vi "CTRE_CANTalonSRX_GetParameter.vi"(8 "error in (no error)":errorcluster, 10 "Parameter":T1=1 items=["Slot 0 - P"=1, "Slot 0 - I"=2, "Slot 0 - D"=3, "Slot 0 - F"=4, "Slot 0 - I Zone"=5, "Slot 0 - Ramp Rate"=6, "Slot 1 - P"=11, "Slot 1 - I"=12, "Slot 1 - D"=13, "Slot 1 - F"=14, "Slot 1 - I Zone"=15, "Slot 1 - Ramp Rate"=16, "Soft Limit - Forward"=21, "Soft Limit - Reverse"=22, "Soft Limit - Forward Enable"=23, "Soft Limit - Reverse Enable"=24, "On Boot - Brake Mode"=31, "On Boot - Limit Normally Closed - Forward"=32, "On Boot - Limit Normally Closed - Reverse"=33, "On Boot - Limit Disabled - Forward"=34, "On Boot - Limit Disabled - Reverse"=35, "Fault - Over Temp"=41, "Fault - Under Voltage"=42, "Fault - Forward Limit"=43, "Fault - Reverse Limit"=44, "Fault - Hardware Failure"=45, "Fault - Forward Soft Limit"=46, "Fault - Reverse Soft Limit"=47, "Sticky Fault - Over Temp"=48, "Sticky Fault - Under Voltage"=49, "Sticky Fault - Forward Limit"=50, "Sticky Fault - Reverse Limit"=51, "Sticky Fault - Forward Soft Limit"=52, "Sticky Fault - Reverse Soft Limit"=53, "Applied Throttle"=61, "Closed-Loop Error"=62, "Select Feedback Device"=63, "Reverse Closed-Loop Output"=64, "Mode Select"=65, "Profile Slot Select"=66, "Ramp Throttle"=67, "Reverse Feedback Sensor"=68, "Limit Switch Enabled"=69, "Limit Switch Closed - Forward"=70, "Limit Switch Closed - Reverse"=71, "Sensor Position"=73, "Sensor Velocity"=74, "Current"=75, "Brake is Enabled"=76, "Encoder Position"=77, "Encoder Velocity"=78, "Encoder Index Rise Events"=79, "Encoder A Pin State"=80, "Encoder B Pin State"=81, "Encoder Index Pin State"=82, "Analog In with Overflow"=83, "Analog In Velocity"=84, "Temperature"=85, "Battery Voltage"=86, "Reset Count"=87, "Reset Flags"=88, "Firmware Version"=89, "Settings Changed"=90, "Quad Filter Enable"=91, "Ignore Disable Broadcast"=92, "I Accumulator"=93, "Status 1 Frame Rate Ms"=94, "Status 2 Frame Rate Ms"=95, "Status 3 Frame Rate Ms"=96, "Status 4 Frame Rate Ms"=97, "Status 6 Frame Rate Ms"=98, "Status 7 Frame Rate Ms"=99, "Enable Index Pin Clear Position"=100, "Peak Positive Output"=104, "Nominal Positive Output"=105, "Peak Negative Output"=106, "Nominal Negative Output"=107, "Quad Index Pin Polarity"=108, "Status 8 Frame Rate Ms"=109, "Allow Position Overflow"=110, "Slot 0 - Allowable Closed-Loop Error"=111, "Number Potentiometer Turns"=112, "Encoder Codes Per Rev"=113, "Pulse Width Decoded Position"=114, "Analog Position"=115, "Voltage Compensation Rate (V/s)"=116, "Slot 1 - Allowable Closed-Loop Error"=117, "Motion Profile Has Underrun Err"=119, "Reserved 120"=120, "Legacy Control Mode"=121, "Motion Magic Acceleration"=122, "Motion Magic Cruise Velocity"=123, "Status 10 Frame Rate"=124, "Current Limit Threshold"=125, "CustomParam0"=137, "CustomParam1"=138, "PersStorageSaving"=139, "ClearPositionOnLimitF"=144, "ClearPositionOnLimitR"=145, "NominalBatteryVoltage"=146, "SampleVelocityPeriod"=147, "SampleVelocityWindow"=148], 11 "CAN Talon SRX Ref":T2={"DeviceStatus"={"status"=FALSE, "code"=0, "source"=""}, "Type"=enum."PWM", "PWM"={"PWM Channel"=enum."PWM 1", "DeadBand"={"Name"="", "maxPositivePwm"=0, "minPositivePwm"=0, "centerPwm"=0, "maxNegativePwm"=0, "minNegativePwm"=0, "angularRange"=0}}, "CAN"={"Device Number"=0, "SetOutput VI Ref"=variant(enum8{"Percent VBus", "Current", "Speed", "Position", "Voltage"} enum."Percent VBus"), "GetOutput VI Ref"=variant(refnum<k1> refnum), "Enable VI Ref"=variant(dbl 12.0), "Disable VI Ref"=variant(enum8{"Percent VBus", "Speed", "Position", "Slave", "Unchanged / Invalid", "Voltage Compensation", "Current", "Motion Profile"} enum."Percent VBus"), "Data"=variant}, "Invert"=FALSE}) -> (0 "error out":errorcluster, 1 "Value Received?":bool, 2 "Parameter Value":dbl, 3 "CAN Talon SRX Ref":T2={"DeviceStatus"={"status"=FALSE, "code"=0, "source"=""}, "Type"=enum."PWM", "PWM"={"PWM Channel"=enum."Invalid", "DeadBand"={"Name"="", "maxPositivePwm"=0, "minPositivePwm"=0, "centerPwm"=0, "maxNegativePwm"=0, "minNegativePwm"=0, "angularRange"=0}}, "CAN"={"Device Number"=0, "SetOutput VI Ref"=variant, "GetOutput VI Ref"=variant, "Enable VI Ref"=variant, "Disable VI Ref"=variant, "Data"=variant}, "Invert"=FALSE})   [LabVIEW 2016]
uses:
  <vilib>/Rock Robotics/WPI/MotorControl/WPI_MotorControlDeviceRef.ctl
  <vilib>/Rock Robotics/WPI/MotorControl/WPI_MotorControlType.ctl
  <vilib>/Rock Robotics/SystemInterfaces/DIO/FPGA_DIOPWMChannel.ctl
  <vilib>/Rock Robotics/WPI/PWM/WPI_PWMDeadband.ctl
  <vilib>/Rock Robotics/WPI/ThirdParty/CanMotor/TalonSRX/WPI_CANTalonSRX_Params.ctl
  <vilib>/Rock Robotics/WPI/ThirdParty/CanMotor/TalonSRX/WPI_CANTalonSRX_MessageIDs.ctl
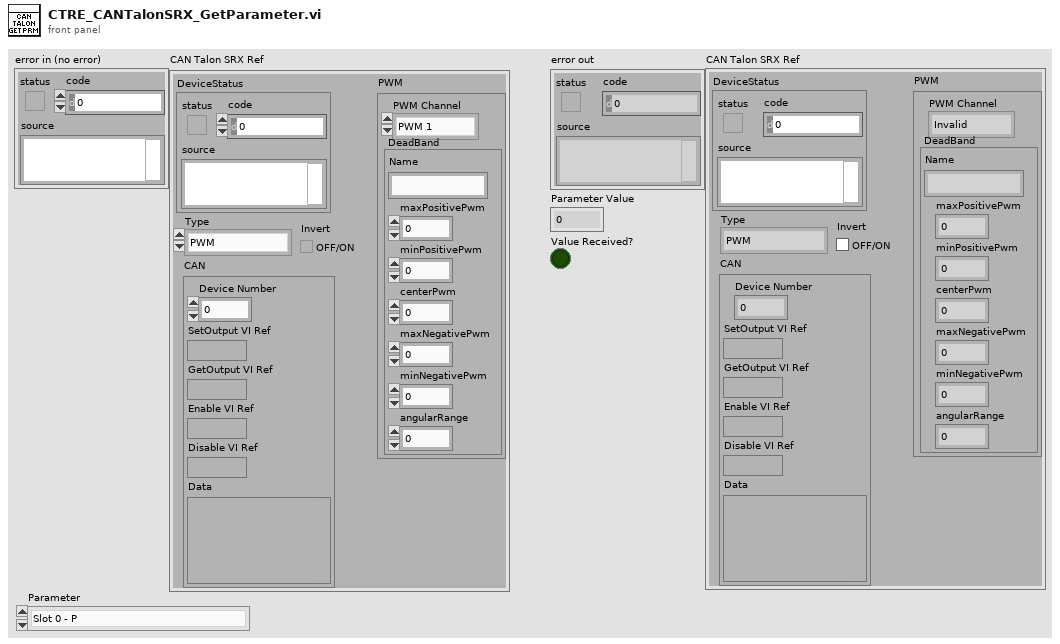
[diagram p1: front panel]
types:
  T1 = typedef "WPI_CANTalonSRX_Params.ctl" = u8
  T2 = typedef "WPI_MotorControlDeviceRef.ctl" = cluster{"DeviceStatus":errorcluster, "Type":T3, "PWM":cluster{"PWM Channel":T4, "DeadBand":T5}, "CAN":cluster{"Device Number":u8, "SetOutput VI Ref":variant, "GetOutput VI Ref":variant, "Enable VI Ref":variant, "Disable VI Ref":variant, "Data":variant}, "Invert":bool}
  T3 = typedef "WPI_MotorControlType.ctl" = enum16{"PWM", "CAN"}
  T4 = typedef "FPGA_DIOPWMChannel.ctl" = enum8{"PWM 0", "PWM 1", "PWM 2", "PWM 3", "PWM 4", "PWM 5", "PWM 6", "PWM 7", "PWM 8", "PWM 9", "PWM MXP 0", "PWM MXP 1", "PWM MXP 2", "PWM MXP 3", "PWM MXP 4", "PWM MXP 5", "PWM MXP 6", "PWM MXP 7", "PWM MXP 8", "PWM MXP 9", "Invalid"}
  T5 = typedef "WPI_PWMDeadband.ctl" = cluster{"Name":string, "maxPositivePwm":i32, "minPositivePwm":i32, "centerPwm":i32, "maxNegativePwm":i32, "minNegativePwm":i32, "angularRange":u16}
  T6 = typedef "WPI_CANTalonSRX_MessageIDs.ctl" = u32
  T7 = cluster{"Message ID":u32, "Timestamp":u32, "Data":u8[]}[]
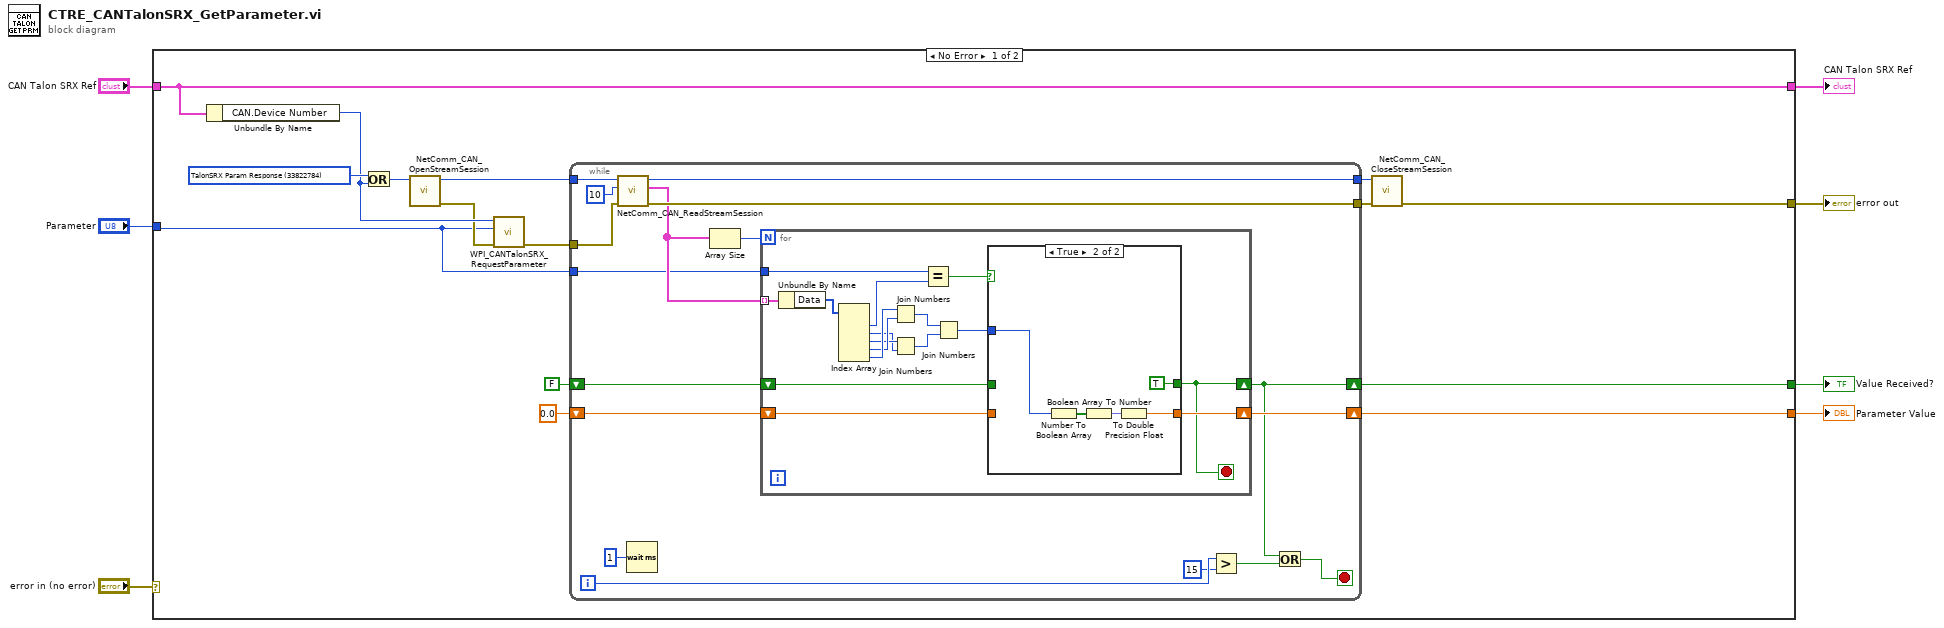
[diagram p0: block diagram]
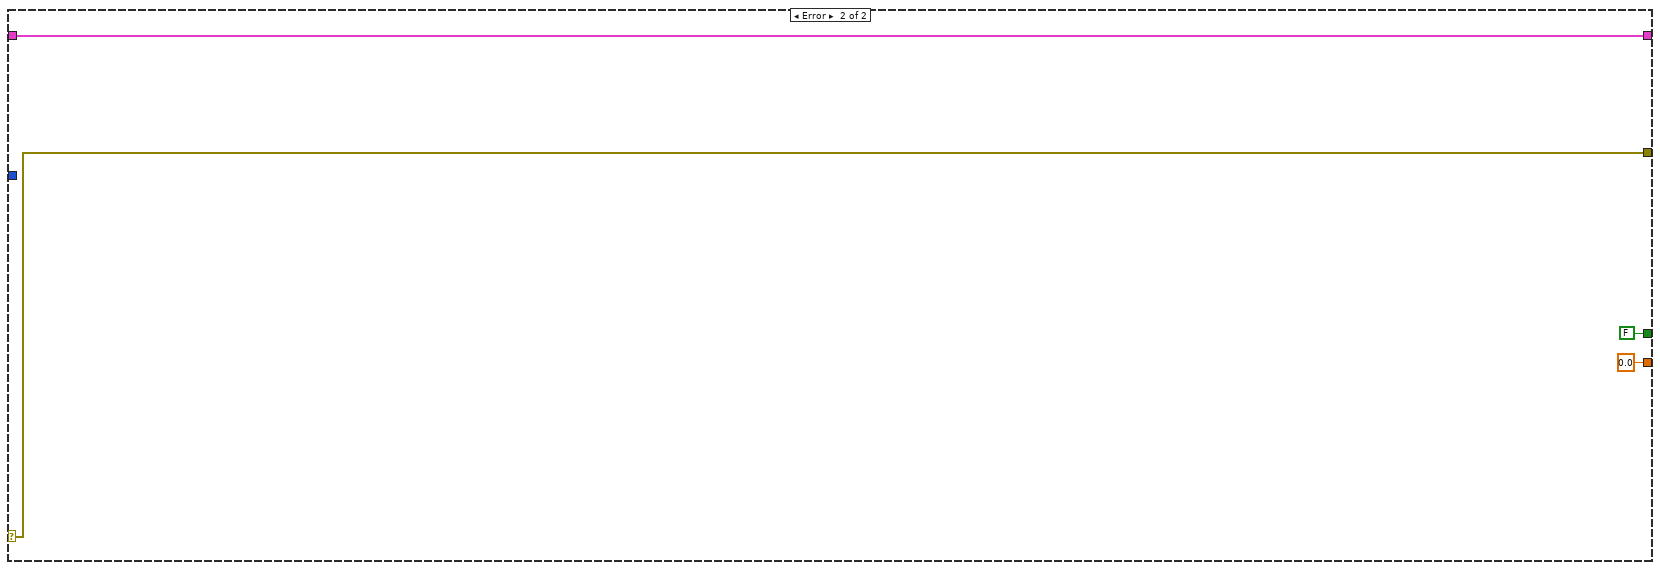
[diagram p3: hidden frame]
diagram:
  n1 = case shown="No Error" "error in (no error)" {
    selector: "error in (no error)" -> [_ w65]
    tunnel: "CAN Talon SRX Ref" -> [w11 w66]
    tunnel: [w12 w65] -> w5
    tunnel: [w11 w66] -> w3
    tunnel: [w10 0.0 ("Numeric")] -> w4
    tunnel: "Parameter" -> [w8 _]
    tunnel: [w9 FALSE] -> w1
    frame No Error {
      w21 = T6 33822784 items=["TalonSRX Control General 10ms"=33816576, "TalonSRX Control Rates Slow"=33816640, "TalonSRX Control ClearFlags Slow"=33816704, "TalonSRX Status General 10ms"=33821696, "TalonSRX Status Feedback 20ms"=33821760, "TalonSRX Status Enc 100ms"=33821824, "TalonSRX Status AinTempVbat 100ms"=33821888, "TalonSRX Status Startup Once"=33821952, "TalonSRX Status Debug"=33822080, "TalonSRX Config SetGainsSlot0 A"=33823808, "TalonSRX Config SetGainsSlot0 B"=33823872, "TalonSRX Config SetGainsSlot1 A"=33823936, "TalonSRX Config SetGainsSlot1 B"=33824000, "TalonSRX Config SetSoftLimits"=33824064, "TalonSRX Config WebControl"=33824128, "TalonSRX Param Request"=33822720, "TalonSRX Param Response"=33822784, "TalonSRX Param Set"=33822848]
      n2 = Unbundle By Name(w11) -> ("CAN.Device Number"=w20:u8)
      n3 = Or(x=w21, y=w20) -> (x .or. y?=w22:T6)
      n4 = call <vilib>:"NetComm_CAN_OpenStreamSession.vi"("Message ID"=w22) -> ("error out"=w18:errorcluster, "Session Handle"=w19:u32)  [unwired: 9 in]
      n5 = call <vilib>:"WPI_CANTalonSRX_RequestParameter.vi"("error in (no error)"=w18, "Parameter"=w8, "Device ID (0)"=w20) -> ("error out"=w17:errorcluster)  [unwired: 7 in, 1 out]
      n6 = while {
        tunnel: w19 -> [w25]
        tunnel: w17 -> [w35]
        shift-right: [w30] -> w9
        shift-left: FALSE -> [w33]
        shift-right: [w31] -> w10
        shift-left: 0.0 ("Numeric") -> [w32]
        tunnel: [w38] -> w14
        tunnel: [w24] -> w13
        tunnel: w8 -> [w23]
        i -> [w28]
        stop <- w29 stop-if-true
        n7 = call <vilib>:"NetComm_CAN_ReadStreamSession.vi"("error in (no error)"=w35, "Messages To Read"=u32 10, "Session Handle"=w25) -> ("error out"=w38:errorcluster, "Messages"=w34:T7, "Session Handle Out"=w24:u32)  [unwired: 6 in]
        n8 = Wait (ms)(milliseconds to wait=u32 1) -> ()  [unwired: 1 out]
        n9 = Array Size(array=w34) -> (size(s)=w36:i32)
        n10 = for {
          N: w36 -> [_]
          tunnel: w34 -> [w55] mode=indexing
          shift-right: [w44] -> w30
          shift-left: w33 -> [w47]
          shift-right: [w45] -> w31
          shift-left: w32 -> [w46]
          tunnel: w23 -> [w41]
          stop <- w44 stop-if-true
          n11 = Unbundle By Name(w55) -> ("Data"=w48:u8[])
          n12 = Index Array(array=w48) -> (element #1=w42:u8, element #2=w49:u8, element #3=w50:u8, element #4=w53:u8, element #5=w54:u8)  [unwired: 5 in]
          n13 = Join Numbers(hi=w54, lo=w53) -> ((hi.lo)=w52:u16)
          n14 = Join Numbers(hi=w50, lo=w49) -> ((hi.lo)=w51:u16)
          n15 = Equal?(x=w41, y=w42) -> (x = y?=w40:bool)
          n16 = Join Numbers(hi=w52, lo=w51) -> ((hi.lo)=w43:u32)
          n17 = case shown="True" w40 {
            tunnel: [w57 TRUE] -> w44
            tunnel: w47 -> [w57 _]
            tunnel: [w56 w58] -> w45
            tunnel: w46 -> [w56 _]
            tunnel: w43 -> [_ w59]
            frame False {
            }
            frame True {
              n18 = Number To Boolean Array(number=w59) -> (Boolean array=w61:bool[])
              n19 = Boolean Array To Number(Boolean array=w61) -> (number=w60:fxp<+,32,10>)
              n20 = To Double Precision Float(number=w60) -> (double precision float=w58:dbl)
            }
          }
        }
        n21 = Greater?(x=w28, y=15) -> (0:w26:bool)
        n22 = Or(x=w30, y=w26) -> (x .or. y?=w29:bool)
      }
      n23 = call <vilib>:"NetComm_CAN_CloseStreamSession.vi"("error in (no error)"=w14, "Session Handle"=w13) -> ("error out"=w12:errorcluster)  [unwired: 9 in]
    }
    frame Error {
    }
  }
  "error out" <- w5
  "Parameter Value" <- w4
  "CAN Talon SRX Ref" <- w3
  "Value Received?" <- w1
